vi "simple tag.vi"() -> ()   [LabVIEW 2017]
uses:
  <vilib>/Skyline/Tag/Shared/typedefs/DataType.ctl
  <vilib>/Skyline/Tag/Wrapper/Wrapper AMQP_class/NI Skyline Tag Wrapper AMQP.lvclass
  C:/Program Files (x86)/National Instruments/LabVIEW 2017/vi.lib/Skyline/Tag/Wrapper/Wrapper_class/NI Skyline Tag Wrapper.lvclass
  <vilib>/Message/Message (Sync).lvclass
  C:/Program Files (x86)/National Instruments/LabVIEW 2017/vi.lib/Message/Message.lvclass
  <vilib>/Skyline/Tag/Wrapper/Wrapper AMQP_class/Open Tag AMQP.vi
  <vilib>/Skyline/Tag/Wrapper/Wrapper_class/Write Tag (Double).vi
  <vilib>/Message/sync/Open (Sync).vi
  <vilib>/Skyline/Tag/Wrapper/Wrapper_class/NI Skyline Tag Wrapper.lvclass
  <vilib>/Skyline/Tag/Shared/NI Skyline Tag.lvlib
  <vilib>/Message/Message.lvclass
panel:
  out "error out 2":errorcluster caption="error out"
  out "error out":errorcluster
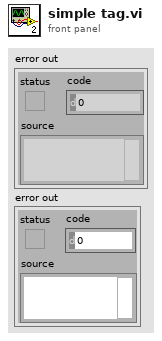
[diagram p1: front panel]
types:
  T1 = typedef "NI Skyline Tag.lvlib/DataType.ctl" = enum32{"Double", "Integer", "String"}
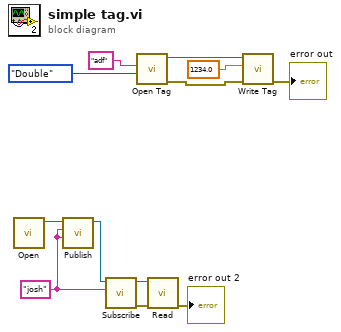
[diagram p0: block diagram]
diagram:
  w5 = "josh" ("topic")
  n1 = call-poly <vilib>:"Open.vi"() -> ("message sync out"=w8:refnum<class "Message (Sync).lvclass">)  [unwired: 10 in, 1 out]
  n2 = call <vilib>:"Publish.vi"("message"=w5, "topic"=w5, "message in"=w8) -> ("message out"=w6:refnum<class "Message (Sync).lvclass">)  [unwired: 7 in, 1 out]
  n3 = call-dynamic "Subscribe.vi"("topic"=w5, "message sync in"=w6) -> ("error out"=w2:errorcluster, "message sync out"=w7:refnum<class "Message (Sync).lvclass">)  [unwired: 8 in]
  n4 = call-poly <vilib>:"Open Tag.vi"("Data Type"=DataType."Double", "Tag Path"="adf") -> ("error out"=w1:errorcluster, "NI Skyline Tag AMQP"=w12:refnum<class "NI Skyline Tag Wrapper AMQP.lvclass">)  [unwired: 8 in]
  n5 = call <vilib>:"Read.vi"("error in (no error)"=w2, "message sync in"=w7) -> ("error out"=→"error out 2":errorcluster)  [unwired: 5 in, 4 out]
  n6 = call-poly <vilib>:"Write Tag.vi"("error in (no error)"=w1, "Value"=1234.0, "NI Skyline Wrapper API in"=w12) -> ("error out"=→"error out":errorcluster)  [unwired: 7 in, 1 out]
